vi "XIPIN_AXI_Direct_Memory_Access_7_1.vi"   [LabVIEW 2017]
doc: "The Xilinx AXI DMA LogiCORE provides a flexible interface for transferring packet data between system memory (AXI4) and AXI4-Stream target IP. Optional Scatter / Gather Engine provides offloading of processor management of DMA transfers. Optional Scatter / Gather Descriptor Queuing allows prefetching of transfer descriptors providing uninterrupted transfer requests to be processed by the primary DMA controllers. Independent operation between MM2S (transmit channel) and S2MM (receive channel) allows for full duplex operation of the AXI DMA engine. Multi-Descriptor per packet functionality is also provided allowing for packet data to be read or written across distributed buffer locations in system memory. Optional AXI4 Control Stream and AXI4 Status Stream provide side band transfer capabilities for transferring user meta data associated with the primary packet transfer. Typical applications for the Control and Status streams are for functions like Checksum offloading on AXI Ethernet. Optional Data Re-Alignment Engines allow for transfers to and from any byte offset in system memory. Simple DMA mode is also provide for a low resource utilization option for commanding simple DMA transfers.\n------------------------------------\n<b>Need License</b> : No\n<b>Interface</b> : AXI4 AXI4-Stream"
uses:
  <vilib>/rvi/XilinxIP/XIPIN_XNode/niFpgaXIPIN.xnode
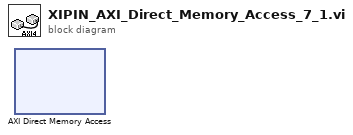
[diagram p0: block diagram]
diagram:
  n1 = xnode ("AXI Direct Memory Access")() -> ()
